vi "LinearQuadraticRegulator_GetK.vi"(11 "in LinearQuadraticRegulator":T2) -> (3 "K":T1)   [LabVIEW 2019, in "Trajectory_Library.lvlib"]
doc: "Returns the controller matrix K.\n \nInput:\n - LinearQuadraticRegulator -- controller data cluster\n\nOutputs:\n - K -- the controller matrix K."
uses:
  Trajectory_Library.lvlib
  <vilib>/Analysis/Matrix/Datatypes/RealMatrix.ctl
  <vilib>/Analysis/Matrix/NI_Matrix.lvlib
  TypeDef/LINEAR_QUADRATIC_REGULATOR.ctl
panel:
  # "Ref State <States,1>"
  # "Comp and capped \noutput <Inputs,1>"
  # "Controller gain\n<Inputs,States>"
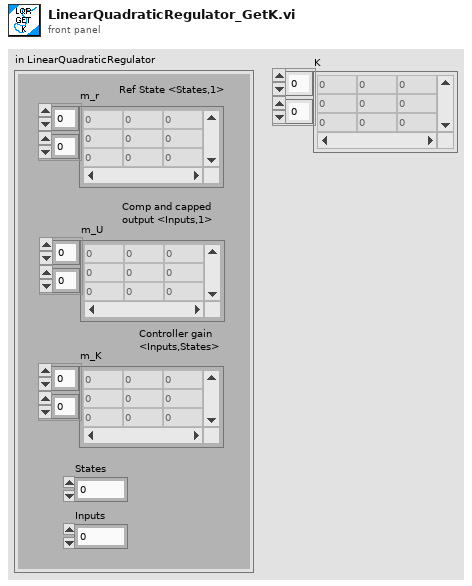
[diagram p1: front panel]
types:
  T1 = typedef "NI_Matrix.lvlib/RealMatrix.ctl" = dbl[][]
  T2 = typedef "Trajectory_Library.lvlib/LINEAR_QUADRATIC_REGULATOR.ctl" = cluster{"m_r":T1, "m_U":T1, "m_K":T1, "States":i32, "Inputs":i32}
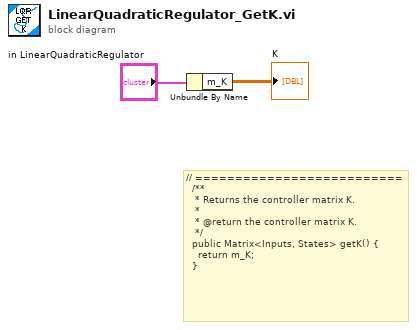
[diagram p0: block diagram]
diagram:
  # "// ==========================\n  /**\n   * Returns the controller matrix K.\n   *\n   * @return the controller matrix K.\n   */\n  public Matrix<Inputs, States> getK() {\n    return m_K;\n  }"
  n1 = Unbundle By Name("in LinearQuadraticRegulator") -> ("m_K"=→"K":T1)
